vi "AVI saves prototyping.vi"() -> ()   [LabVIEW 2017]
uses:
  Typedefs/Frame Size.ctl
  <vilib>/vision/Avi.llb/IMAQ AVI2 Codec Path.ctl
  <vilib>/vision/Image Controls.llb/IMAQ Image.ctl
panel:
  in  "GreenImageArray":T1[](array[typedef])=["remote image 0000000015F6793C", "remote image 0000000015F679A4", "remote image 0000000015F67A0C", "remote image 0000000015F67A74", "remote image 0000000015F67ADC", "remote image 0000000015F67B44", "remote image 0000000015F67BAC"]
  out "x = y?":bool[][][](array[boolean])
  out "OK":bool
  out "Image":T1(plugin-control)
  in  "Experiment folder path":path=path "C:/Users/Teo/Desktop/New folder"
  out "Bit Depth":u32
  out "min value":dbl
  out "max value":dbl
  out "output array":dbl[][](array[numeric])
  out "?":i32
  out "Codec Used":string
  in  "Frames to grab":i32=7
  in  "stop":bool
  in  "Quality":i32=750
  in  "Codex index":i32
  out "Codec Names":string[](array[string])
  in  "AVI File Path":path=path "C:/Users/Teo/Desktop/test.avi"
  in  "Rate (Hz)":u32=10
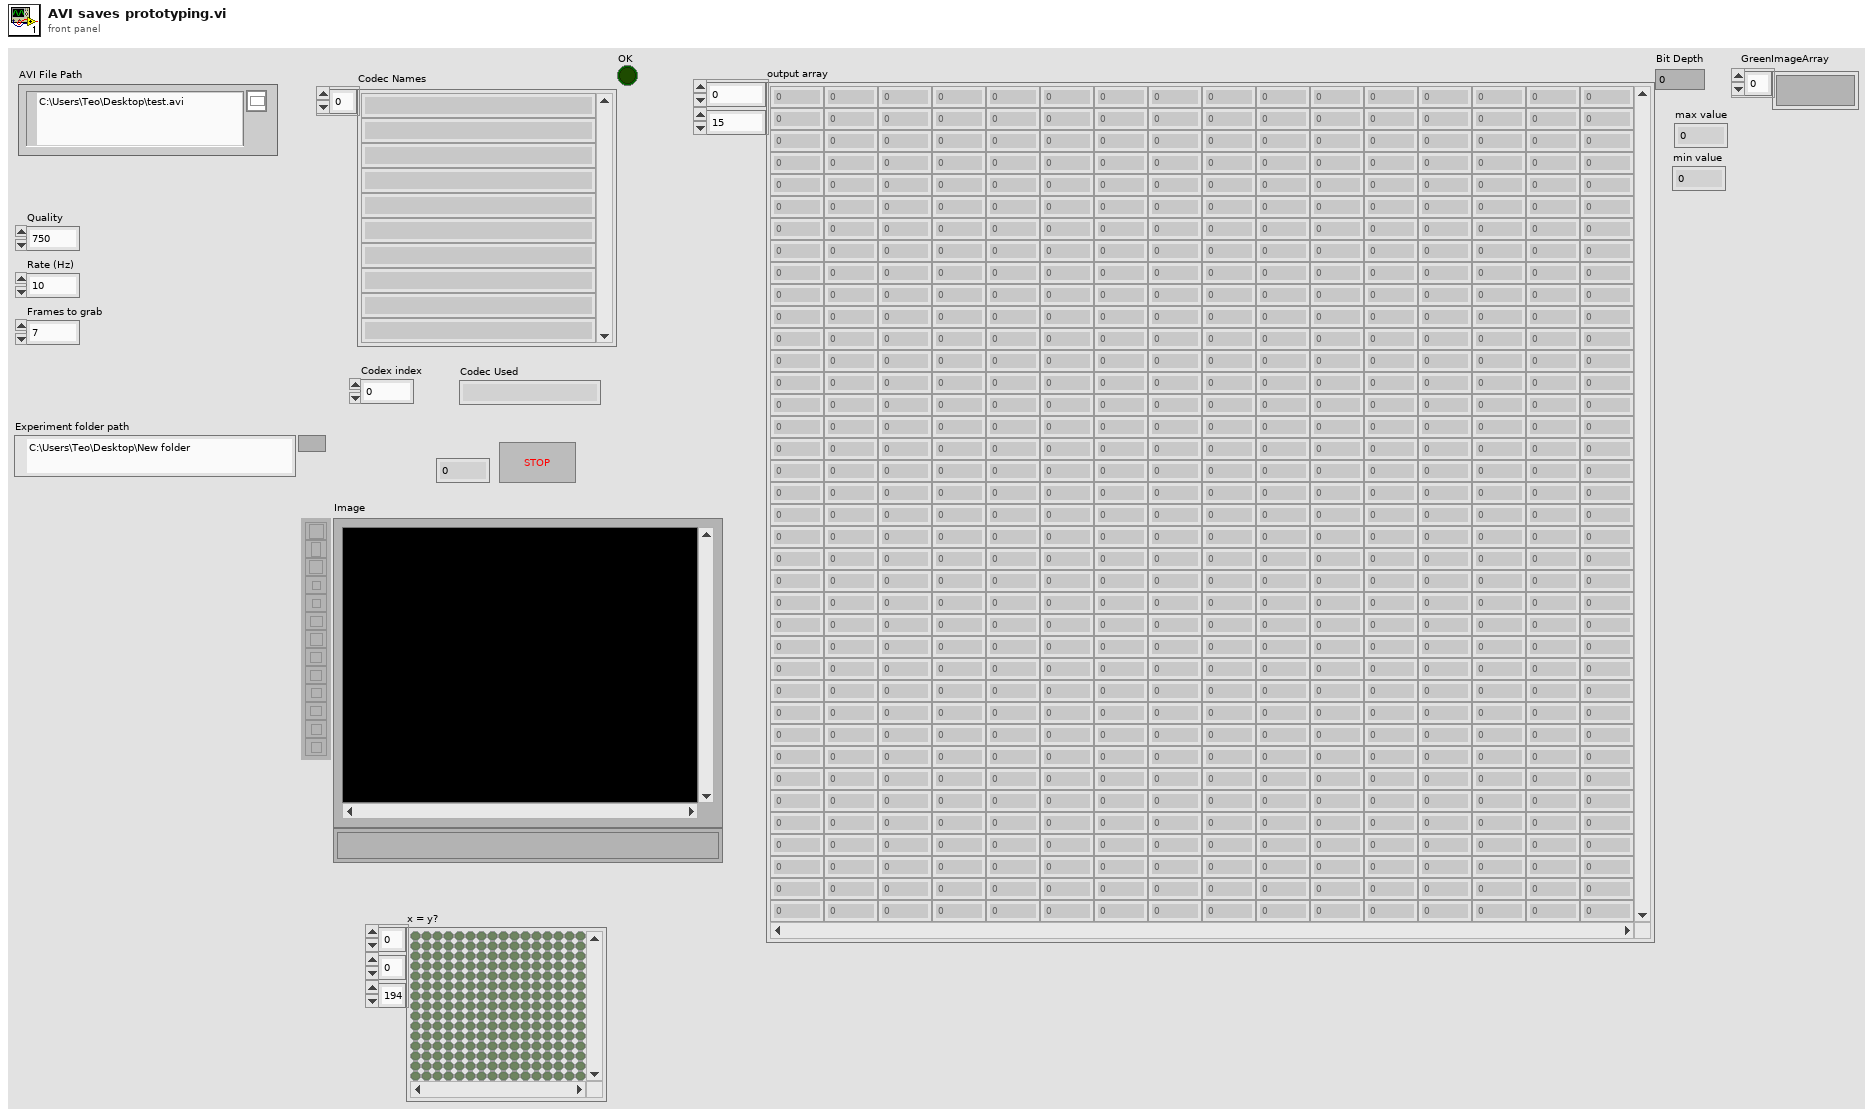
[diagram p1: front panel]
types:
  T1 = typedef "IMAQ Image.ctl" = refnum<image>
  T2 = typedef "Image Type" = u32
  T3 = typedef "IMAQ AVI2 Codec Path.ctl" = u32
  T4 = typedef "IMAQ AVI2 Refnum.ctl" = refnum<k20>
  T5 = typedef "Frame Size.ctl" = u16
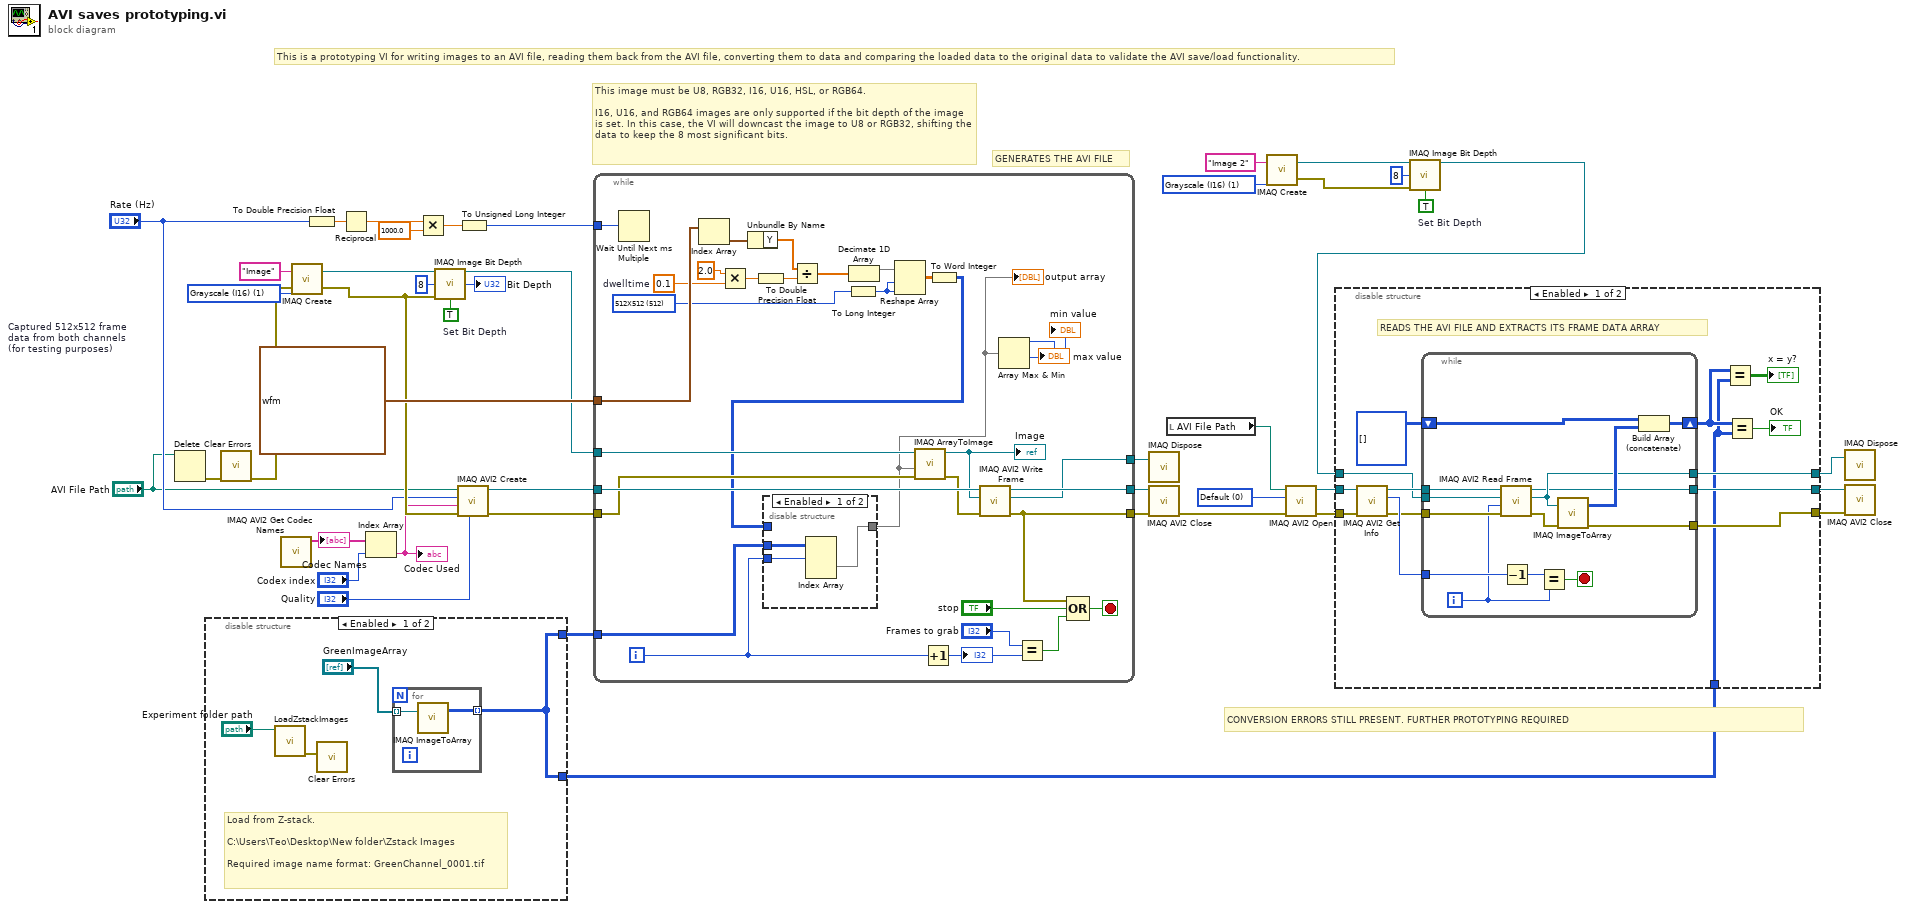
[diagram p0: block diagram]
diagram:
  w6 = TRUE  # Set Bit Depth
  w2 = T2 1 items=["Grayscale (U8)", "Grayscale (I16)", "Grayscale (SGL)", "Complex (CSG)", "RGB (U32)", "HSL (U32)", "RGB (U64)", "Grayscale (U16)"] ("Image Type")
  w16 = T3 0 items=["Default", "System", "Built in Vision"] ("Codec Source")
  w29 = TRUE  # Set Bit Depth
  w33 = T2 1 items=["Grayscale (U8)", "Grayscale (I16)", "Grayscale (SGL)", "Complex (CSG)", "RGB (U32)", "HSL (U32)", "RGB (U64)", "Grayscale (U16)"] ("Image Type")
  w44 = waveform(dbl)[] [{"t0"=timestamp(0 s since 1904-01-01), "dt"=1.0, "Y"=array[524288 elements]}]  # Captured 512x512 frame data from both channels (for testing purposes)
  # "CONVERSION ERRORS STILL PRESENT. FURTHER PROTOTYPING REQUIRED"
  # "This is a prototyping VI for writing images to an AVI file, reading them back from the AVI file, converting them to data and comparing the loaded data to the original data to validate the AVI save/load functionality."
  # "GENERATES THE AVI FILE"
  # "This image must be U8, RGB32, I16, U16, HSL, or RGB64. \n\nI16, U16, and RGB64 images are only supported if the bit depth of the image is set. In this case, the VI will downcast the image to U8 or RGB32, shifting the data to keep the 8 most significant bits."
  n1 = Delete(path (use dialog)="AVI File Path") -> (error out=w11:errorcluster)  [unwired: 4 in, 2 out]
  n2 = disable-structure shown="Enabled" {
    disable-tunnel: [w45 _] -> w26
    disable-tunnel: [w45 _] -> w23
    frame Enabled {
      # "Load from Z-stack.\n\nC:\\Users\\Teo\\Desktop\\New folder\\Zstack Images\n\nRequired image name format: GreenChannel_0001.tif"
      n3 = call "LoadZstackImages.vi"("Experiment folder path"="Experiment folder path") -> ("Error Out"=w46:errorcluster)  [unwired: 3 in, 7 out]
      n4 = call <vilib>:"Clear Errors.vi"("error in (no error)"=w46) -> ()  [unwired: 5 in, 2 out]
      n5 = for {
        tunnel: "GreenImageArray" -> [w50] mode=indexing
        tunnel: [w49] -> w45 mode=indexing
        n6 = call "IMAQ ImageToArray"("Image"=w50) -> ("Image Pixels (I16)"=w49:i16[][])  [unwired: 3 in, 4 out]
      }
    }
    frame Disabled {
    }
  }
  n7 = call <vilib>:"Clear Errors.vi"("error in (no error)"=w11) -> ("error out"=w9:errorcluster)  [unwired: 5 in, 1 out]
  n8 = call "IMAQ AVI2 Get Codec Names"() -> ("Codec Names"=w39:string[])  [unwired: 10 in, 1 out]
  "Codec Names" <- w39
  n9 = call "IMAQ Create"("Image Name"="Image", "Image Type"=w33, "error in (no error)"=w9) -> ("New Image"=w31:T1, "error out"=w27:errorcluster)  [unwired: 2 in]
  n10 = To Double Precision Float(number="Rate (Hz)") -> (double precision float=w35:dbl)
  n11 = Reciprocal(x=w35) -> (1/x=w43:dbl)
  n12 = Index Array(array=w39, index="Codex index") -> (element=w24:string)
  "Codec Used" <- w24
  n13 = Multiply(x=w43, y=1000.0) -> (x*y=w41:dbl)
  n14 = call "IMAQ Image Bit Depth"("Image"=w31, "Bit Depth (0)"=u32 8, "error in (no error)"=w27, "Get/Set Bit Depth? (Set)"=w29) -> ("Image Out"=w22:T1, "Bit Depth"=→"Bit Depth":u32)  [unwired: 9 in, 1 out]
  n15 = call "IMAQ AVI2 Create"("Quality"="Quality", "error in (no error)"=w27, "Codec"=w24, "Frames Per Second"="Rate (Hz)", "AVI Path"="AVI File Path") -> ("error out"=w36:errorcluster, "AVI Refnum"=w37:T4)  [unwired: 5 in]
  n16 = To Unsigned Long Integer(number=w41) -> (unsigned 32bit integer=w34:u32)
  n17 = while {
    tunnel: w44 -> [w68]
    tunnel: w34 -> [w82]
    tunnel: w37 -> [w79]
    tunnel: w36 -> [w59]
    tunnel: [w78] -> w18
    tunnel: [w77] -> w17
    tunnel: [w63] -> w8
    tunnel: w22 -> [w62]
    tunnel: w26 -> [w55]
    i -> [w54]
    stop <- w81 stop-if-true
    w67 = 0.1  # dwelltime
    w65 = T5 512 items=["20X20"=0, "100X100"=100, "128X128"=128, "200X200"=200, "256X256"=256, "512X512"=512] ("Frame Size")
    n18 = Wait Until Next ms Multiple(millisecond multiple=w82) -> ()  [unwired: 1 out]
    n19 = Index Array(array=w68) -> (element=w73:waveform(dbl))  [unwired: 1 in]
    n20 = Multiply(x=2.0, y=w67) -> (x*y=w71:dbl)
    n21 = Unbundle By Name ("Get Waveform Components")(w73) -> ("Y"=w70:dbl[])
    n22 = To Double Precision Float(number=w71) -> (double precision float=w74:dbl)
    n23 = Divide(x=w70, y=w74) -> (x/y=w69:dbl[])
    n24 = To Long Integer(number=w65) -> (32bit integer=w64:i32)
    n25 = Decimate 1D Array(w69) -> (w66:dbl[])  [unwired: 1 out]
    n26 = Reshape Array(w66, w64, w64) -> (w57:dbl[][])
    n27 = Increment(x=w54) -> (x+1=w76:i32)
    "?" <- w76
    n28 = To Word Integer(number=w57) -> (16bit integer=w53:i16[][])
    n29 = disable-structure shown="Enabled" {
      disable-tunnel: w55 -> [w85 _]
      disable-tunnel: w54 -> [w84 _]
      disable-tunnel: [w83 w86] -> w52
      disable-tunnel: w53 -> [_ w86]
      frame Enabled {
        n30 = Index Array(array=w85, index (dim 0)=w84) -> (element=w83:i16[][])  [unwired: 2 in]
      }
      frame Disabled {
      }
    }
    "output array" <- w52
    n31 = call "IMAQ ArrayToImage"("error in (no error)"=w59, "Image Pixels (I16)"=w52, "Image"=w62) -> ("error out"=w58:errorcluster, "Image Out"=w51:T1)  [unwired: 7 in]
    "Image" <- w51
    n32 = call "IMAQ AVI2 Write Frame"("error in (no error)"=w58, "Image"=w51, "AVI Refnum"=w79) -> ("error out"=w77:errorcluster, "Image Out (duplicate)"=w63:T1, "AVI Refnum (duplicate)"=w78:T4)  [unwired: 6 in]
    n33 = Array Max & Min(array=w52) -> (max value=→"max value":i16, min value=→"min value":i16)  [unwired: 2 out]
    n34 = Equal?(x="Frames to grab", y=w76) -> (x = y?=w56:bool)
    n35 = Compound Arithmetic op=OR(w77, "stop", w56) -> (w81:bool)
  }
  n36 = call "IMAQ Dispose"("Image"=w8) -> ()  [unwired: 2 in, 4 out]
  n37 = call "IMAQ AVI2 Close"("error in (no error)"=w17, "AVI Refnum"=w18) -> ("error out"=w12:errorcluster)  [unwired: 9 in]
  n38 = local read "AVI File Path"() -> (w14:path)
  n39 = call "IMAQ Create"("Image Name"="Image 2", "Image Type"=w2) -> ("New Image"=w4:T1, "error out"=w7:errorcluster)  [unwired: 3 in]
  n40 = call "IMAQ AVI2 Open"("error in (no error)"=w12, "Codec Source"=w16, "AVI File Path"=w14) -> ("error out"=w13:errorcluster, "AVI Refnum"=w15:T4)  [unwired: 7 in]
  n41 = call "IMAQ Image Bit Depth"("Image"=w4, "Bit Depth (0)"=u32 8, "error in (no error)"=w7, "Get/Set Bit Depth? (Set)"=w6) -> ("Image Out"=w1:T1)  [unwired: 9 in, 2 out]
  n42 = disable-structure shown="Enabled" {
    disable-tunnel: w23 -> [w88 _]
    disable-tunnel: w1 -> [w95 w115]
    disable-tunnel: w15 -> [w94 w117]
    disable-tunnel: w13 -> [w93 w116]
    disable-tunnel: [w91 w117] -> w21
    disable-tunnel: [w90 w116] -> w20
    disable-tunnel: [w92 w115] -> w19
    frame Enabled {
      # "READS THE AVI FILE AND EXTRACTS ITS FRAME DATA ARRAY"
      n43 = call "IMAQ AVI2 Get Info"("error in (no error)"=w93, "AVI Refnum"=w94) -> ("error out"=w98:errorcluster, "Number of Frames"=w100:u32, "AVI Refnum (duplicate)"=w99:T4)  [unwired: 5 in, 2 out]
      n44 = while {
        tunnel: w100 -> [w114]
        tunnel: w99 -> [w112]
        tunnel: w98 -> [w111]
        tunnel: w95 -> [w110]
        shift-right: [w108] -> w89
        shift-left: i16[][][] [] -> [w107]
        tunnel: [w106] -> w92
        tunnel: [w105] -> w91
        tunnel: [w103] -> w90
        i -> [w102]
        stop <- w113 stop-if-true
        n45 = call "IMAQ AVI2 Read Frame"("error in (no error)"=w111, "Frame Number"=w102, "Image"=w110, "AVI Refnum"=w112) -> ("error out"=w104:errorcluster, "Image Out"=w106:T1, "AVI Refnum (duplicate)"=w105:T4)  [unwired: 5 in]
        n46 = Decrement(x=w114) -> (x-1=w101:u32)
        n47 = Equal?(x=w101, y=w102) -> (x = y?=w113:bool)
        n48 = call "IMAQ ImageToArray"("error in (no error)"=w104, "Image"=w106) -> ("error out"=w103:errorcluster, "Image Pixels (I16)"=w109:i16[][])  [unwired: 2 in, 3 out]
        n49 = Build Array (concatenate)(w107, w109) -> (w108:i16[][][])
      }
      n50 = Equal?(x=w89, y=w88) -> (x = y?=→"x = y?":bool[][][])
      n51 = Equal?(x=w89, y=w88) -> (x = y?=→"OK":bool)
    }
    frame Disabled {
    }
  }
  n52 = call "IMAQ Dispose"("Image"=w19) -> ()  [unwired: 2 in, 4 out]
  n53 = call "IMAQ AVI2 Close"("error in (no error)"=w20, "AVI Refnum"=w21) -> ()  [unwired: 9 in, 1 out]
